vi "AutoData.vi"(8 "error in (no error)":errorcluster) -> (0 "error out":errorcluster, 3 "AutoData":T3)   [LabVIEW 2013]
uses:
  HotGoalDetectType.ctl
  AutoMode.ctl
  AutoData.ctl
panel:
  in  "Defaults":enum32{"General", "Drive", "Hot Goal", "Shoot"}(tab)
  in  "EndInLowGear?":bool=TRUE
  in  "HotGoalTypeDefault":T1
  in  "StartInLowGear?":bool=TRUE
  in  "BallSettleWait":u32=130
  in  "PreCheckGoalWait":u32=260
  in  "AutoDefaultMode":T2
  in  "DriveMinTime":u32=2000
  in  "DriveDistance":dbl=36.0 format="%#_13g"
  in  "DriveTimeout":u32=4000
  in  "DriveBackWait":u32=1000
  in  "DriveBackSpeed":dbl=-1.0
  in  "AccelBackward":dbl=0.1
  in  "AccelForward":dbl=0.1
  in  "SlowdownDistance":dbl=36.0 format="%#_13g"
  in  "BrakeDistance":dbl=12.0 format="%#_13g"
  in  "PreScumbagWait":u32
  in  "StartShootTime":u32=5000
  in  "AutoIDKey":i32=3061
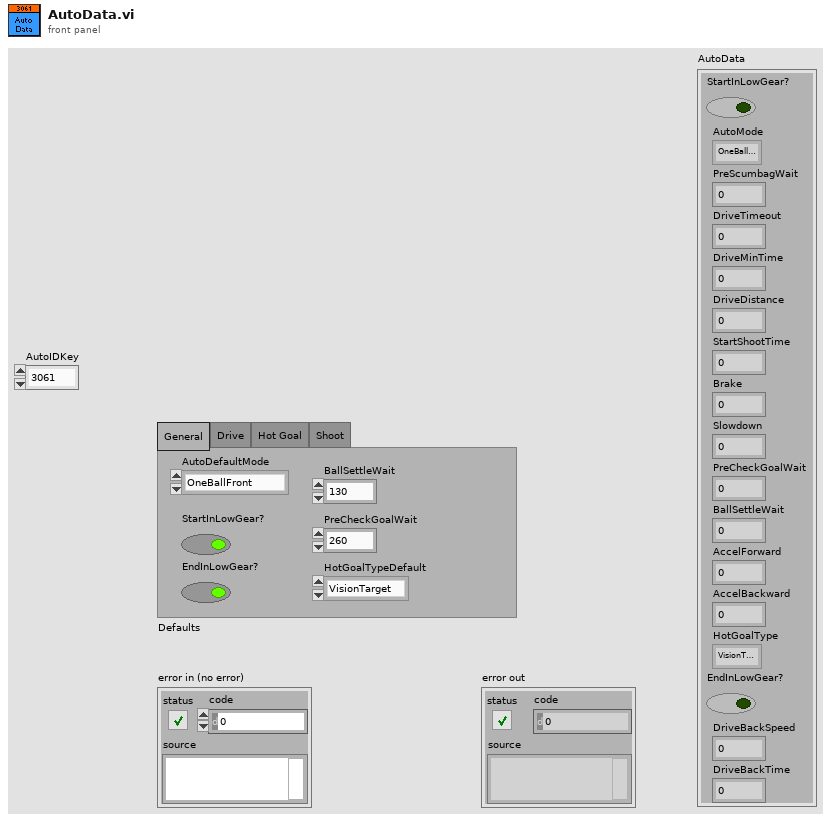
[diagram p1: front panel]
types:
  T1 = typedef "HotGoalDetectType.ctl" = enum16{"VisionTarget", "Kinect", "SoundDetect", "Webcam"}
  T2 = typedef "AutoMode.ctl" = enum16{"OneBallFront", "OneBallCollector", "TwoBallNormal", "TwoBallHot"}
  T3 = typedef "AutoData.ctl" = cluster{"StartInLowGear?":bool, "AutoMode":T2, "PreScumbagWait":u32, "DriveTimeout":u32, "DriveMinTime":u32, "DriveDistance":dbl, "StartShootTime":u32, "Brake":dbl, "Slowdown":dbl, "PreCheckGoalWait":u32, "BallSettleWait":u32, "AccelForward":dbl, "AccelBackward":dbl, "HotGoalType":T1, "EndInLowGear?":bool, "DriveBackSpeed":dbl, "DriveBackTime":u32}
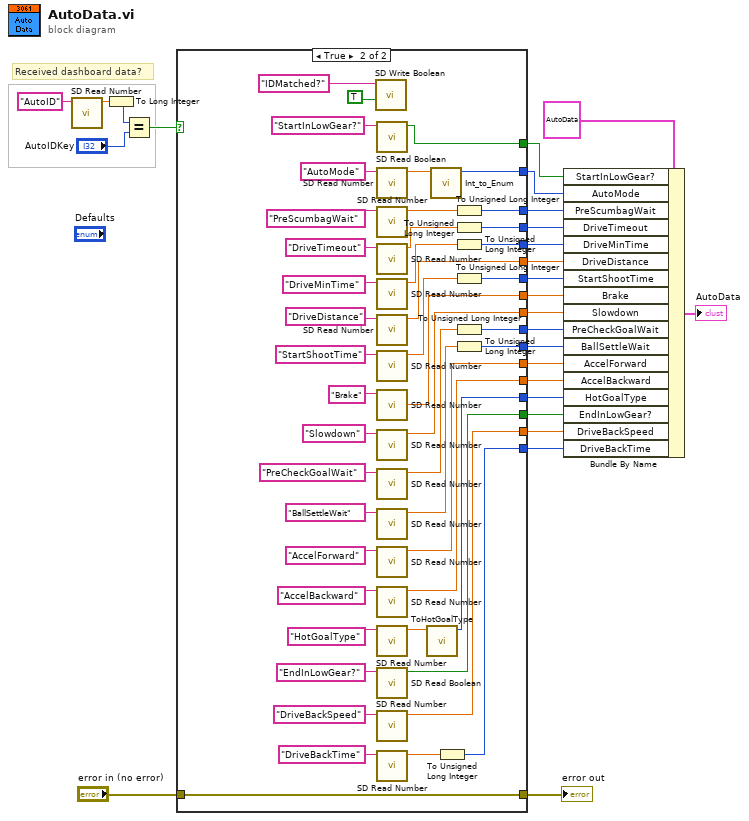
[diagram p0: block diagram]
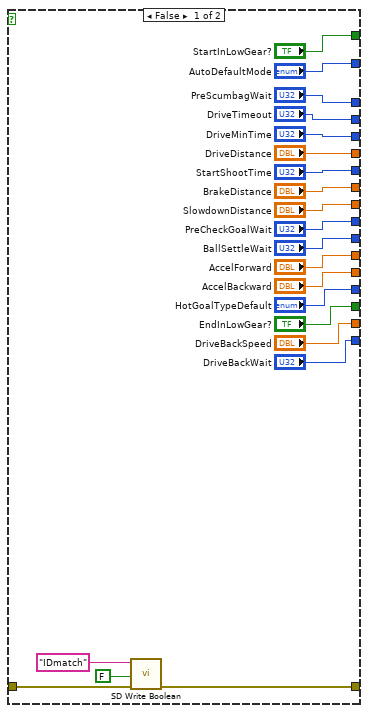
[diagram p2: hidden frame]
diagram:
  # "Received dashboard data?"
  n1 = call <vilib>:"SD Read Number.vi"("Name"="AutoID") -> ("Numeric"=w26:dbl)  [unwired: 8 in, 2 out]
  n2 = To Long Integer(number=w26) -> (32bit integer=w24:i32)
  n3 = Equal?(x=w24, y="AutoIDKey") -> (x = y?=w22:bool)
  n4 = case shown="True" w22 {
    tunnel: "error in (no error)" -> [w46 w54]
    tunnel: [w45 w54] -> w2
    tunnel: ["AutoDefaultMode" w90] -> w18
    tunnel: ["DriveTimeout" w85] -> w3
    tunnel: ["DriveMinTime" w83] -> w4
    tunnel: ["DriveDistance" w81] -> w5
    tunnel: ["BrakeDistance" w79] -> w7
    tunnel: ["SlowdownDistance" w78] -> w8
    tunnel: ["PreCheckGoalWait" w75] -> w9
    tunnel: ["BallSettleWait" w72] -> w10
    tunnel: ["HotGoalTypeDefault" w68] -> w13
    tunnel: ["StartInLowGear?" w67] -> w19
    tunnel: ["AccelForward" w63] -> w11
    tunnel: ["AccelBackward" w62] -> w12
    tunnel: ["EndInLowGear?" w60] -> w14
    tunnel: ["DriveBackSpeed" w58] -> w15
    tunnel: ["DriveBackWait" w55] -> w16
    tunnel: ["StartShootTime" w51] -> w6
    tunnel: ["PreScumbagWait" w48] -> w17
    frame False {
      n5 = call <vilib>:"SD Write Boolean.vi"("error in"=w46, "Boolean"=FALSE, "Name"="IDmatch") -> ("error out"=w45:errorcluster)  [unwired: 7 in, 1 out]
    }
    frame True {
      n6 = call <vilib>:"SD Write Boolean.vi"("Boolean"=TRUE, "Name"="IDMatched?") -> ()  [unwired: 8 in, 2 out]
      n7 = call <vilib>:"SD Read Boolean.vi"("Name"="StartInLowGear?") -> ("Boolean"=w67:bool)  [unwired: 8 in, 2 out]
      n8 = call <vilib>:"SD Read Number.vi"("Name"="AutoMode") -> ("Numeric"=w91:dbl)  [unwired: 8 in, 2 out]
      n9 = call <vilib>:"SD Read Number.vi"("Name"="PreScumbagWait") -> ("Numeric"=w50:dbl)  [unwired: 8 in, 2 out]
      n10 = call <vilib>:"SD Read Number.vi"("Name"="DriveTimeout") -> ("Numeric"=w84:dbl)  [unwired: 8 in, 2 out]
      n11 = call <vilib>:"SD Read Number.vi"("Name"="DriveMinTime") -> ("Numeric"=w82:dbl)  [unwired: 8 in, 2 out]
      n12 = call <vilib>:"SD Read Number.vi"("Name"="DriveDistance") -> ("Numeric"=w81:dbl)  [unwired: 8 in, 2 out]
      n13 = call <vilib>:"SD Read Number.vi"("Name"="StartShootTime") -> ("Numeric"=w53:dbl)  [unwired: 8 in, 2 out]
      n14 = call <vilib>:"SD Read Number.vi"("Name"="Brake") -> ("Numeric"=w79:dbl)  [unwired: 8 in, 2 out]
      n15 = call <vilib>:"SD Read Number.vi"("Name"="Slowdown") -> ("Numeric"=w78:dbl)  [unwired: 8 in, 2 out]
      n16 = call <vilib>:"SD Read Number.vi"("Name"="PreCheckGoalWait") -> ("Numeric"=w74:dbl)  [unwired: 8 in, 2 out]
      n17 = call <vilib>:"SD Read Number.vi"("Name"="BallSettleWait") -> ("Numeric"=w71:dbl)  [unwired: 8 in, 2 out]
      n18 = call <vilib>:"SD Read Number.vi"("Name"="AccelForward") -> ("Numeric"=w63:dbl)  [unwired: 8 in, 2 out]
      n19 = call <vilib>:"SD Read Number.vi"("Name"="AccelBackward") -> ("Numeric"=w62:dbl)  [unwired: 8 in, 2 out]
      n20 = call <vilib>:"SD Read Number.vi"("Name"="HotGoalType") -> ("Numeric"=w69:dbl)  [unwired: 8 in, 2 out]
      n21 = call <vilib>:"SD Read Boolean.vi"("Name"="EndInLowGear?") -> ("Boolean"=w60:bool)  [unwired: 8 in, 2 out]
      n22 = call <vilib>:"SD Read Number.vi"("Name"="DriveBackSpeed") -> ("Numeric"=w58:dbl)  [unwired: 8 in, 2 out]
      n23 = call <vilib>:"SD Read Number.vi"("Name"="DriveBackTime") -> ("Numeric"=w57:dbl)  [unwired: 8 in, 2 out]
      n24 = call "ToHotGoalType.vi"("IntIn"=w69) -> ("EnumOut"=w68:T1)  [unwired: 10 in]
      n25 = call "Int_to_Enum.vi"("IntIn"=w91) -> ("EnumOut"=w90:T2)  [unwired: 10 in]
      n26 = To Unsigned Long Integer(number=w57) -> (unsigned 32bit integer=w55:u32)
      n27 = To Unsigned Long Integer(number=w50) -> (unsigned 32bit integer=w48:u32)
      n28 = To Unsigned Long Integer(number=w84) -> (unsigned 32bit integer=w85:u32)
      n29 = To Unsigned Long Integer(number=w82) -> (unsigned 32bit integer=w83:u32)
      n30 = To Unsigned Long Integer(number=w53) -> (unsigned 32bit integer=w51:u32)
      n31 = To Unsigned Long Integer(number=w74) -> (unsigned 32bit integer=w75:u32)
      n32 = To Unsigned Long Integer(number=w71) -> (unsigned 32bit integer=w72:u32)
    }
  }
  "error out" <- w2
  n33 = Bundle By Name(cluster=T3 {"StartInLowGear?"=FALSE, "AutoMode"=enum."OneBallFront", "PreScumbagWait"=0, "DriveTimeout"=0, "DriveMinTime"=0, "DriveDistance"=0.0, "StartShootTime"=0, "Brake"=0.0, "Slowdown"=0.0, "PreCheckGoalWait"=0, "BallSettleWait"=0, "AccelForward"=0.0, "AccelBackward"=0.0, "HotGoalType"=enum."VisionTarget", "EndInLowGear?"=FALSE, "DriveBackSpeed"=0.0, "DriveBackTime"=0} ("AutoData"), "StartInLowGear?"=w19, "AutoMode"=w18, "PreScumbagWait"=w17, "DriveTimeout"=w3, "DriveMinTime"=w4, "DriveDistance"=w5, "StartShootTime"=w6, "Brake"=w7, "Slowdown"=w8, "PreCheckGoalWait"=w9, "BallSettleWait"=w10, "AccelForward"=w11, "AccelBackward"=w12, "HotGoalType"=w13, "EndInLowGear?"=w14, "DriveBackSpeed"=w15, "DriveBackTime"=w16) -> (→"AutoData":T3)
